vi "Post Build Script (Powershell build).vi"(8 "Package Source Folder":path=path "C:/user/patrick/git/Multichannel-Lockin/src", 9 "Package Version":string="2.8.9.18", 10 "Product Name":string="Multichannel Lockin", 11 "Output Package File Path":path) -> (0 "error out":errorcluster)   [LabVIEW 2019, in "PostBuildSupport.lvclass"]
doc: "After you manually build the Application and Installer inside your project, you can then call this VI to create single self-extracting installer file. It is meant to be placed inside \"Post-Build Custom Action.vi\" that is called post VIPM package build."
uses:
  PostBuildSupport.lvclass
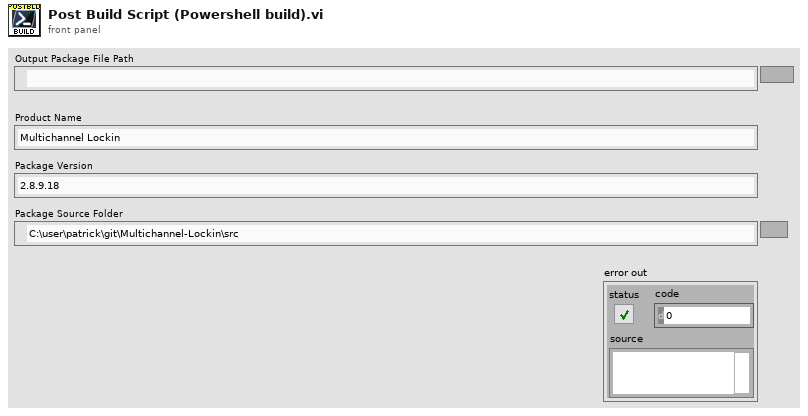
[diagram p1: front panel]
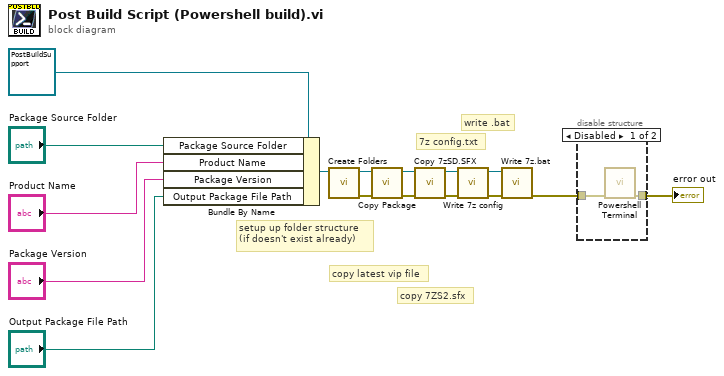
[diagram p0: block diagram]
diagram:
  # "copy 7ZS2.sfx"
  # "setup up folder structure \n(if doesn't exist already)"
  # "copy latest vip file"
  # "7z config.txt"
  # "write .bat"
  n1 = Bundle By Name(cluster=refnum<class "PostBuildSupport.lvclass"> refnum ("PostBuildSupport in"), "Package Source Folder"="Package Source Folder", "Product Name"="Product Name", "Package Version"="Package Version", "Output Package File Path"="Output Package File Path") -> (w10:refnum<class "PostBuildSupport.lvclass">)
  n2 = call "Create Folders.vi"("PostBuildSupport in"=w10) -> ("error out"=w7:errorcluster, "PostBuildSupport out"=w12:refnum<class "PostBuildSupport.lvclass">)  [unwired: 9 in]
  n3 = call "Copy Package.vi"("error in (no error)"=w7, "PostBuildSupport in"=w12) -> ("error out"=w6:errorcluster, "PostBuildSupport out"=w11:refnum<class "PostBuildSupport.lvclass">)  [unwired: 8 in]
  n4 = call "Copy 7zSD.SFX.vi"("error in (no error)"=w6, "PostBuildSupport in"=w11) -> ("error out"=w8:errorcluster, "PostBuildSupport out"=w9:refnum<class "PostBuildSupport.lvclass">)  [unwired: 8 in]
  n5 = call "Write 7z config.vi"("error in (no error)"=w8, "PostBuildSupport in"=w9) -> ("error out"=w15:errorcluster, "PostBuildSupport out"=w16:refnum<class "PostBuildSupport.lvclass">)  [unwired: 8 in]
  n6 = call "Write 7z.bat.vi"("error in (no error)"=w15, "PostBuildSupport in"=w16) -> ("error out"=w2:errorcluster)  [unwired: 8 in, 1 out]
  n7 = disable-structure shown="Disabled" {
    disable-tunnel: w2 -> [w18 _]
    disable-tunnel: [w17 _] -> w1
    frame Disabled {
      n8 = call "Powershell Terminal.vi"("error in (no error)"=w18) -> ("error out"=w17:errorcluster)  [unwired: 10 in]
    }
    frame Enabled {
    }
  }
  "error out" <- w1
